vi "valve controll.vi"(0 "VISA Refnum in":refnum<visa-resource-name>, 5 "Valve 1":bool, 7 "Valve 2":bool, 9 "Valve 3":bool, 11 "error in (no error)":errorcluster, 12 "Reset valves":bool) -> (4 "VISA Refnum in 2":refnum<visa-resource-name>, 6 "Active Valve":string, 15 "error out":errorcluster)   [LabVIEW 2016]
panel:
  in  "Valve":string="Valve 3"
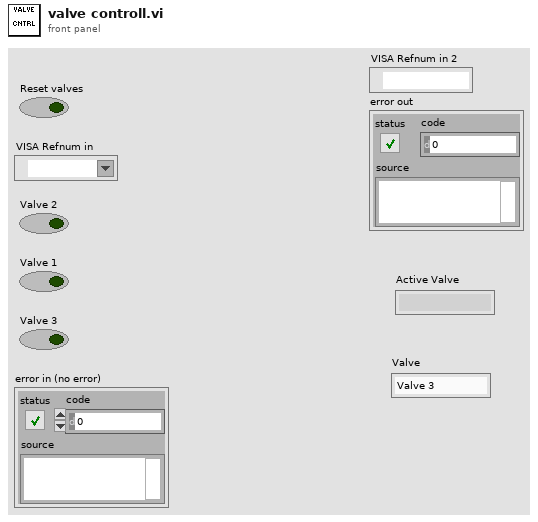
[diagram p1: front panel]
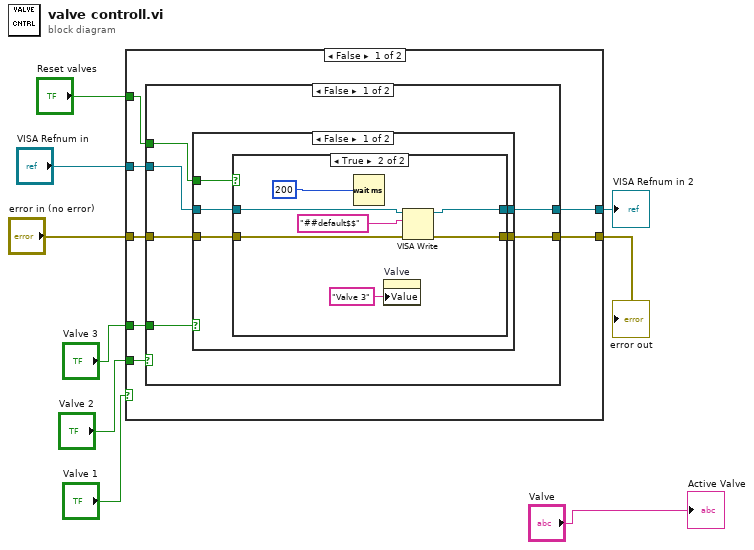
[diagram p0: block diagram]
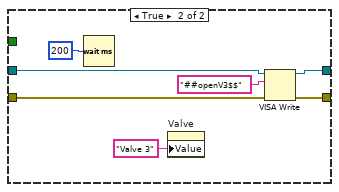
[diagram p3: hidden frame]
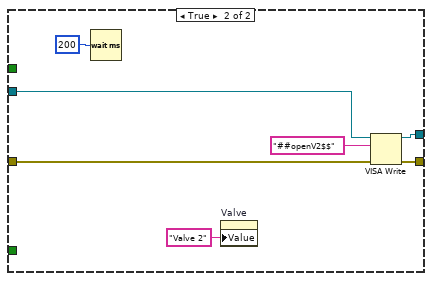
[diagram p4: hidden frame]
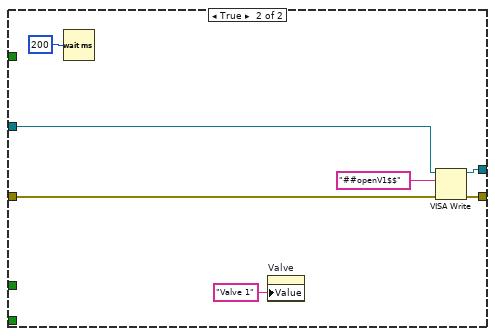
[diagram p5: hidden frame]
diagram:
  n1 = case shown="False" "Valve 1" {
    tunnel: [w15 w55] -> w2
    tunnel: "Valve 2" -> [w14 _]
    tunnel: "Valve 3" -> [w13 _]
    tunnel: "Reset valves" -> [w12 _]
    tunnel: "VISA Refnum in" -> [w11 w53]
    tunnel: "error in (no error)" -> [w10 w52]
    tunnel: [w16 w56] -> w3
    frame False {
      n2 = case shown="False" w14 {
        tunnel: w11 -> [w21 w49]
        tunnel: w10 -> [w20 w48]
        tunnel: [w19 w47] -> w16
        tunnel: [w18 w46] -> w15
        tunnel: w13 -> [w22 _]
        tunnel: w12 -> [w17 _]
        frame False {
          n3 = case shown="False" w22 {
            tunnel: w21 -> [w27 w42]
            tunnel: w20 -> [w26 w41]
            tunnel: [w24 w39] -> w19
            tunnel: [w23 w38] -> w18
            tunnel: w17 -> [w25 _]
            frame False {
              n4 = case shown="True" w25 {
                tunnel: w27 -> [w29 w35]
                tunnel: w26 -> [w28 w34]
                tunnel: [w29 w33] -> w24
                tunnel: [w28 w32] -> w23
                frame False {
                }
                frame True {
                  n5 = Wait (ms)(milliseconds to wait=u32 200) -> ()  [unwired: 1 out]
                  n6 = property on="Valve" class="Str"("Value"="Valve 3" ("Valve")) -> ()  [unwired: 2 in, 2 out]
                  n7 = VISA Write(VISA resource name=w35, write buffer="##default$$", error in (no error)=w34) -> (VISA resource name out=w33:refnum<visa-resource-name>, error out=w32:errorcluster)  [unwired: 1 out]
                }
              }
            }
            frame True {
              n8 = Wait (ms)(milliseconds to wait=u32 200) -> ()  [unwired: 1 out]
              n9 = property on="Valve" class="Str"("Value"="Valve 3" ("Valve")) -> ()  [unwired: 2 in, 2 out]
              n10 = VISA Write(VISA resource name=w42, write buffer="##openV3$$", error in (no error)=w41) -> (VISA resource name out=w39:refnum<visa-resource-name>, error out=w38:errorcluster)  [unwired: 1 out]
            }
          }
        }
        frame True {
          n11 = Wait (ms)(milliseconds to wait=u32 200) -> ()  [unwired: 1 out]
          n12 = property on="Valve" class="Str"("Value"="Valve 2" ("Valve")) -> ()  [unwired: 2 in, 2 out]
          n13 = VISA Write(VISA resource name=w49, write buffer="##openV2$$", error in (no error)=w48) -> (VISA resource name out=w47:refnum<visa-resource-name>, error out=w46:errorcluster)  [unwired: 1 out]
        }
      }
    }
    frame True {
      n14 = Wait (ms)(milliseconds to wait=u32 200) -> ()  [unwired: 1 out]
      n15 = property on="Valve" class="Str"("Value"="Valve 1" ("Valve")) -> ()  [unwired: 2 in, 2 out]
      n16 = VISA Write(VISA resource name=w53, write buffer="##openV1$$", error in (no error)=w52) -> (VISA resource name out=w56:refnum<visa-resource-name>, error out=w55:errorcluster)  [unwired: 1 out]
    }
  }
  "VISA Refnum in 2" <- w3
  "error out" <- w2
  "Active Valve" <- "Valve"
